vi "S2C_GlobalMenus.vi"() -> ()   [LabVIEW 2015]
panel:
  in  "ExcludedDrivers":string[](array[string])=["RMS"]
  in  "MenuRef":refnum<k9>
  in  "Measurement":string[][](array[string])=[["RMS"], ["Envelope Frequency"], ["Peak"], ["Crest Factor"], ["Duty Cycle %"], ["Peak-Peak"], ["Frequency"], ["THD"], ["Positive Peak"], ["Negative Peak"], ["Mag_H1"], ["Phase_H1"], ["Mag_H3"], ["Phase_H3"], ["Mag_H5"], ["Phase_H5"]]
  in  "Analyzer":string[][](array[string])=[["Measure"], ["Clear Waveforms"]]
  in  "LoadBox":string[][](array[string])=[["Set Load"], ["Clear Load"]]
  in  "Drivers":string[][](array[string])
  in  "PathRelays":string[][](array[string])
  in  "FootSwitch":string[][](array[string])
  in  "HandSwitch":string[][](array[string])
  in  "Insert/Extract":string[][](array[string])
  in  "TouchScreen":string[][](array[string])
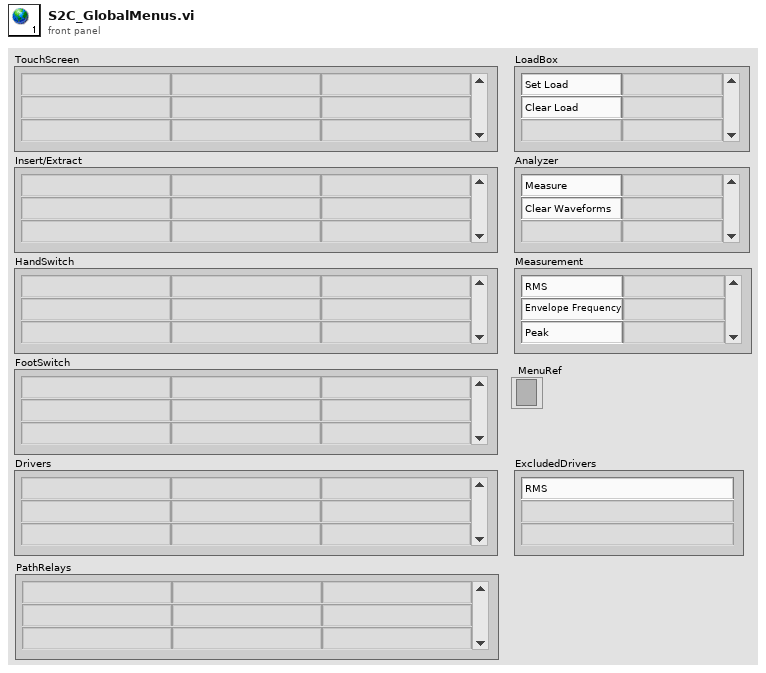
[diagram p1: front panel]
diagram:
